vi "write_params.vi"(8 "error in (no error)":errorcluster caption="entrée d'erreur (pas d'erreur)", 10 "params":T1={"n_components"=2.0, "perplexity"=30.0, "early_exaggeration"=12.0, "learning_rate"=200.0, "n_iter"=1000.0, "n_iter_without_progress"=0.0, "min_grad_norm"=1e-07, "metric"={"metric_type"="euclidean", "metric_function"=""}, "init"={"init_type"="random", "init_list"=[]}, "verbose"=0.0, "random_state"=0.0, "method"="barnes_hut", "angle"=0.5, "n_jobs"=1.0}, 11 "TSNE en entrée":refnum<class "TSNE.lvclass">) -> (0 "error out":errorcluster caption="sortie d'erreur", 3 "TSNE en sortie":refnum<class "TSNE.lvclass">)   [LabVIEW 2020, in "TSNE.lvclass"]
uses:
  TSNE.lvclass
  Controls/tsne_params.ctl
  TSNE.lvclass/TSNE.ctl
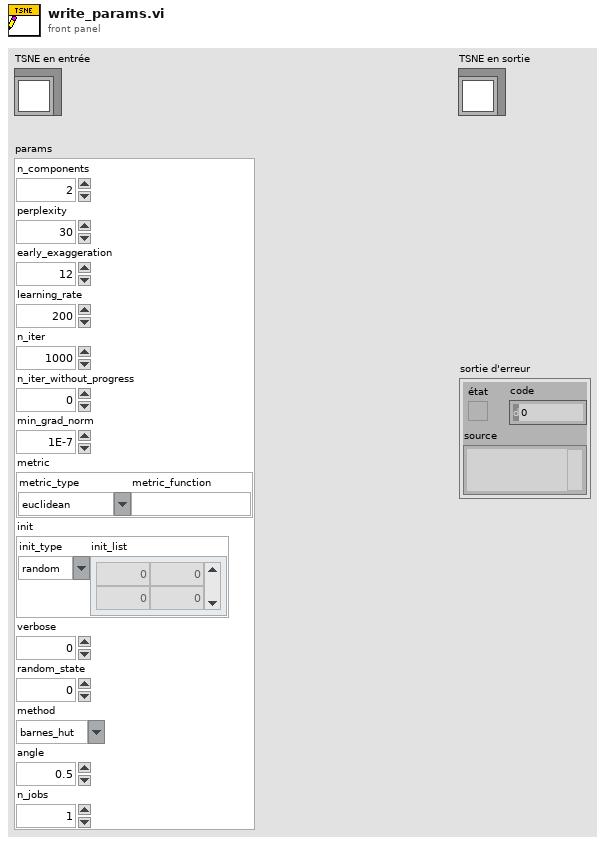
[diagram p1: front panel]
types:
  T1 = typedef "tsne_params.ctl" = cluster{"n_components":dbl, "perplexity":dbl, "early_exaggeration":dbl, "learning_rate":dbl, "n_iter":dbl, "n_iter_without_progress":dbl, "min_grad_norm":dbl, "metric":cluster{"metric_type":string, "metric_function":string}, "init":cluster{"init_type":string, "init_list":dbl[][]}, "verbose":dbl, "random_state":dbl, "method":string, "angle":dbl, "n_jobs":dbl}
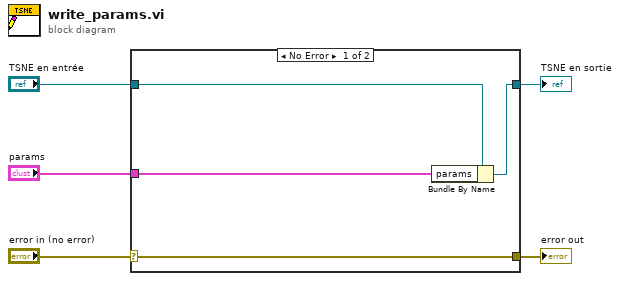
[diagram p0: block diagram]
diagram:
  n1 = case shown="No Error" "error in (no error)" {
    selector: "error in (no error)" -> [w9 w10]
    tunnel: [w9 w10] -> w4
    tunnel: [w7 w11] -> w2
    tunnel: "TSNE en entrée" -> [w8 w11]
    tunnel: "params" -> [w6 _]
    frame No Error {
      n2 = Bundle By Name(cluster=w8, "params"=w6) -> (w7:refnum<class "TSNE.lvclass">)
    }
    frame Error {
    }
  }
  "error out" <- w4
  "TSNE en sortie" <- w2
